vi "Sensores_LabView.vi"() -> ()   [LabVIEW 2014]
uses:
  <vilib>/LabVIEW Interface for Arduino/Type Defs/Board Type.ctl
  <vilib>/LabVIEW Interface for Arduino/Type Defs/Pin Mode.ctl
  <vilib>/LabVIEW Interface for Arduino/LabVIEW Interface for Arduino.lvlib
panel:
  out "Sensor de Movimiento":bool
  out "Sensor de temperatura":dbl(slide) scale=0.0..100.0
  out "Indicador fotoresistencia":dbl(knob) scale=0.0..100.0
  out "Sensor de Movimiento":dbl
  out "Aire acondicionado":bool
  out "Iluminacion":bool
  out "UPS":bool
  out "On / Off":bool
  in  "Iluminacion deseada":dbl
  in  "VISA resource":refnum<visa-resource-name>
  in  "stop":bool
  in  "Temperatura deseada":dbl
  # "Entradas"
  # "Salidas"
  # "Valores deseados"
  # "Información\ndel programa"
  # "Interruptores"
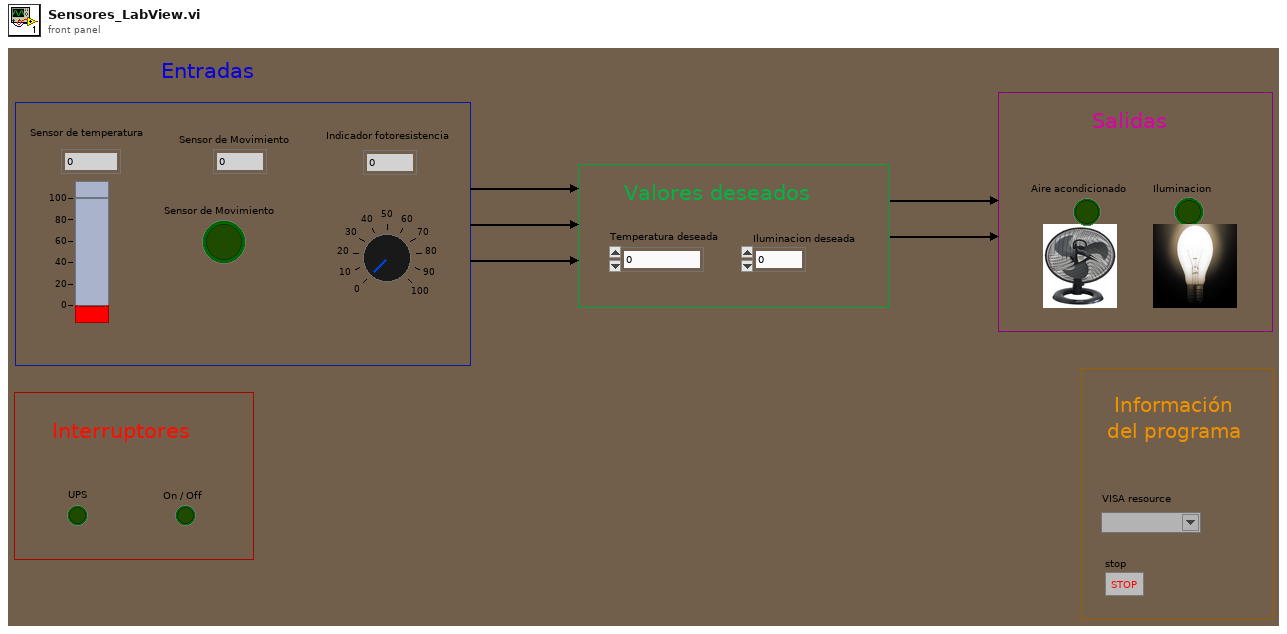
[diagram p1: front panel]
types:
  T1 = typedef "LabVIEW Interface for Arduino.lvlib/Board Type.ctl" = enum16{"Uno", "Dimuelanove w/Atmega 328", "Mega 2560"}
  T2 = typedef "LabVIEW Interface for Arduino.lvlib/Arduino Resource.ctl" = cluster{"VISA resource":refnum<visa-resource-name>, "Board Type":T1, "Connection Type":enum8{"USB / Serial"}, "Bytes Per Packet (15)":u8}
  T3 = typedef "LabVIEW Interface for Arduino.lvlib/Pin Mode.ctl" = enum8{"Input", "Output"}
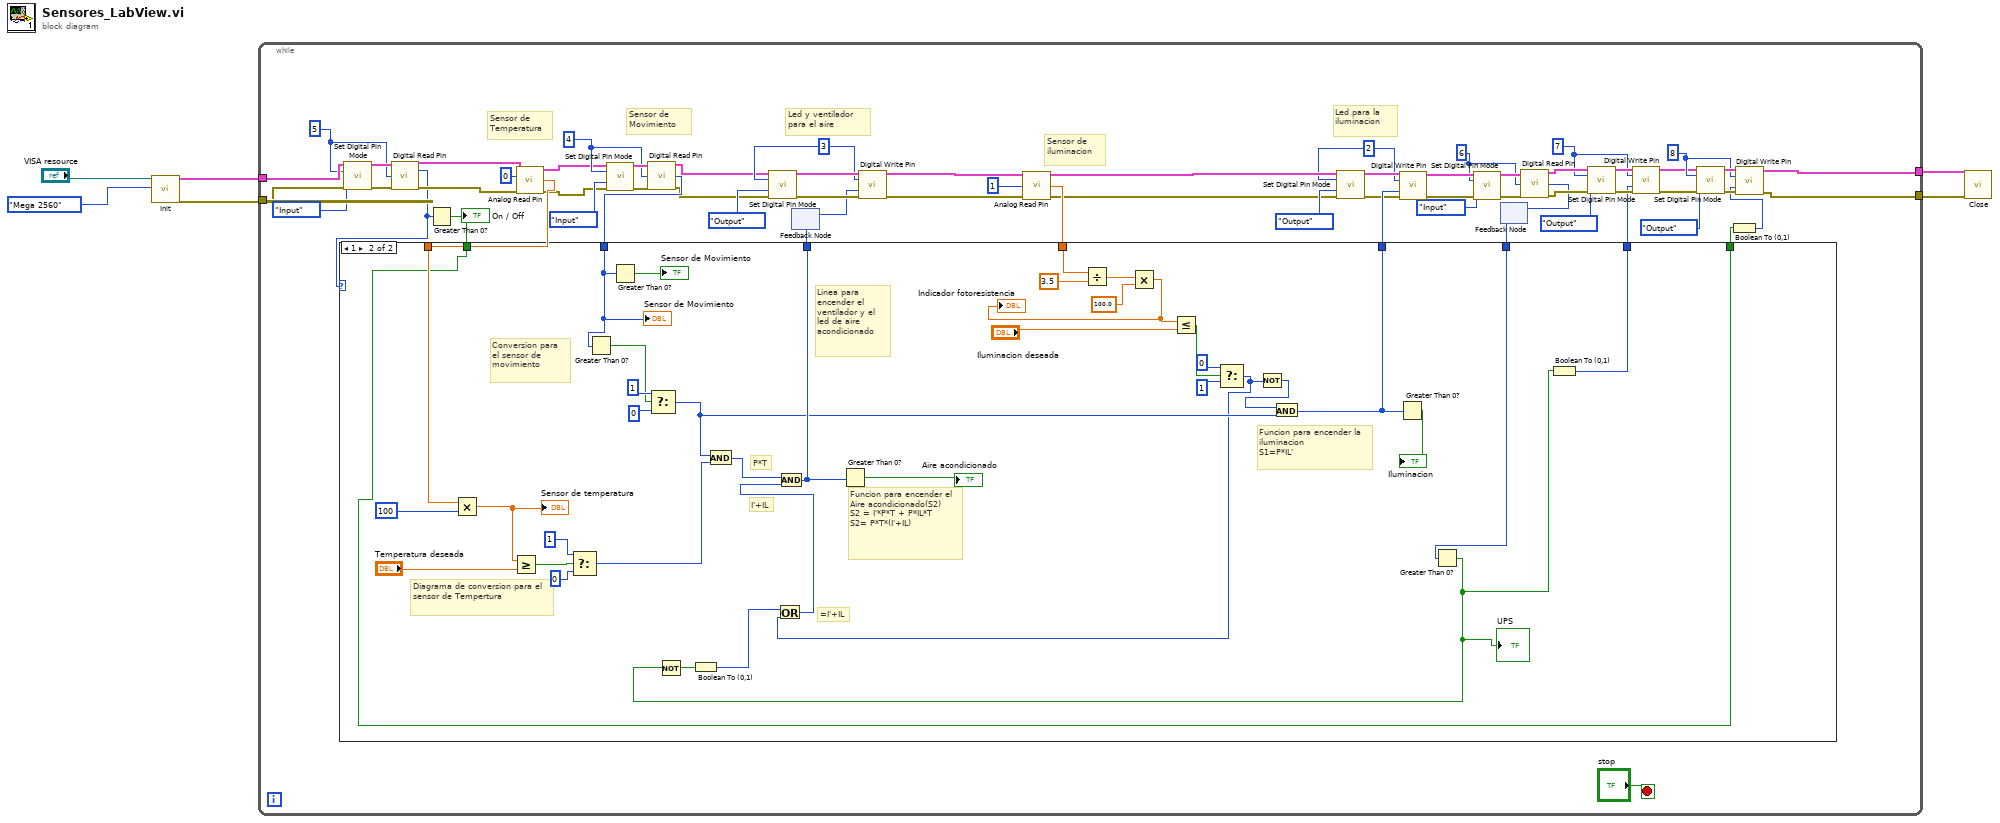
[diagram p0: block diagram]
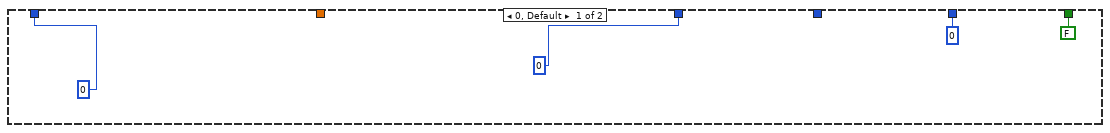
[diagram p2: hidden frame]
diagram:
  n1 = call <vilib>:"Init.vi"("VISA resource"="VISA resource", "Board Type (Uno)"=Board_Type."Mega 2560") -> ("Arduino Resource"=w6:T2, "error out"=w5:errorcluster)  [unwired: 16 in]
  n2 = while {
    tunnel: w6 -> [w37]
    tunnel: w5 -> [w36]
    tunnel: [w10] -> w3
    tunnel: [w9] -> w2
    stop <- "stop" stop-if-true
    w14 = u8 8 ("Digital I/O Pin")
    w19 = u8 7 ("Digital I/O Pin")
    w27 = u8 6 ("Digital I/O Pin")
    w35 = u8 5 ("Digital I/O Pin")
    w45 = u8 4 ("Digital I/O Pin")
    w52 = u8 2 ("Digital I/O Pin")
    w53 = u8 3 ("Digital I/O Pin")
    # "Led para la iluminacion"
    # "Led y ventilador para el aire"
    # "Sensor de Movimiento"
    # "Sensor de iluminacion"
    # "Sensor de Temperatura"
    n3 = call <vilib>:"Set Digital Pin Mode.vi"("Arduino Resource"=w37, "Digital I/O Pin"=w35, "Pin Mode (Input)"=Pin_Mode."Input", "error in"=w36) -> ("Arduino Resource"=w44:T2, "error out"=w43:errorcluster)  [unwired: 10 in]
    n4 = call <vilib>:"Digital Read Pin.vi"("Arduino Resource"=w44, "Digital I/O Pin (0)"=w35, "error in"=w43) -> ("Arduino Resource"=w41:T2, "Value"=w33:u8, "error out"=w38:errorcluster)  [unwired: 10 in]
    n5 = Greater Than 0?(x=w33) -> (x > 0?=w13:bool)
    "On / Off" <- w13
    n6 = call <vilib>:"Analog Read Pin.vi"("Arduino Resource"=w41, "Analog Input Pin (0)"=u8 0, "error in"=w38) -> ("Arduino Resource"=w39:T2, "Voltage"=w70:dbl, "error out"=w40:errorcluster)  [unwired: 10 in]
    n7 = call <vilib>:"Set Digital Pin Mode.vi"("Arduino Resource"=w39, "Digital I/O Pin"=w45, "Pin Mode (Input)"=Pin_Mode."Input", "error in"=w40) -> ("Arduino Resource"=w50:T2, "error out"=w49:errorcluster)  [unwired: 10 in]
    n8 = call <vilib>:"Digital Read Pin.vi"("Arduino Resource"=w50, "Digital I/O Pin (0)"=w45, "error in"=w49) -> ("Arduino Resource"=w47:T2, "Value"=w48:u8, "error out"=w46:errorcluster)  [unwired: 10 in]
    n9 = call <vilib>:"Set Digital Pin Mode.vi"("Arduino Resource"=w47, "Digital I/O Pin"=w53, "Pin Mode (Input)"=Pin_Mode."Output", "error in"=w46) -> ("Arduino Resource"=w65:T2, "error out"=w64:errorcluster)  [unwired: 10 in]
    n10 = feedback #1() -> (w54:i32)  [unwired: 1 in]
    n11 = call <vilib>:"Digital Write Pin.vi"("Arduino Resource"=w65, "Digital I/O Pin (0)"=w53, "Value (0)"=w54, "error in"=w64) -> ("Arduino Resource"=w61:T2, "error out"=w60:errorcluster)  [unwired: 10 in]
    n12 = call <vilib>:"Analog Read Pin.vi"("Arduino Resource"=w61, "Analog Input Pin (0)"=u8 1, "error in"=w60) -> ("Arduino Resource"=w59:T2, "Voltage"=w67:dbl, "error out"=w58:errorcluster)  [unwired: 10 in]
    n13 = call <vilib>:"Set Digital Pin Mode.vi"("Arduino Resource"=w59, "Digital I/O Pin"=w52, "Pin Mode (Input)"=Pin_Mode."Output", "error in"=w58) -> ("Arduino Resource"=w57:T2, "error out"=w56:errorcluster)  [unwired: 10 in]
    n14 = feedback #2() -> (w20:u8)  [unwired: 1 in]
    n15 = case shown="1" w33 {
      tunnel: w70 -> [_ w109]
      tunnel: w67 -> [_ w106]
      tunnel: [0 w86] -> w62
      tunnel: [0 w94] -> w55
      tunnel: w48 -> [_ w76]
      tunnel: w20 -> [_ w83]
      tunnel: [i16 0 w82] -> w18
      tunnel: w13 -> [_ w81]
      tunnel: [FALSE w81] -> w12
      frame 0, Default {
      }
      frame 1 {
        # "Funcion para encender la iluminacion\nS1=P*IL'"
        # "P*T"
        # "I'+IL"
        # "=I'+IL"
        # "Linea para encender el ventilador y el led de aire acondicionado"
        # "Funcion para encender el Aire acondicionado(S2)\nS2 = I'*P*T + P*IL*T \nS2= P*T*(I'+IL)"
        # "Conversion para el sensor de movimiento"
        # "Diagrama de conversion para el sensor de Tempertura"
        n16 = Multiply(x=w109, y=100) -> (x*y=w108:dbl)
        "Sensor de temperatura" <- w108
        n17 = Greater Or Equal?(x=w108, y="Temperatura deseada") -> (x >= y?=w104:bool)
        n18 = Select(t=1, s=w104, f=0) -> (s? t:f=w101:i32)
        n19 = Greater Than 0?(x=w76) -> (x > 0?=w84:bool)
        n20 = Greater Than 0?(x=w76) -> (x > 0?=→"Sensor de Movimiento":bool)
        n21 = Select(t=1, s=w84, f=0) -> (s? t:f=w89:i32)
        n22 = And(x=w89, y=w101) -> (x .and. y?=w96:i32)
        n23 = Divide(x=w106, y=3.5) -> (x/y=w79:dbl)
        n24 = Multiply(x=w79, y=100.0) -> (x*y=w77:dbl)
        "Indicador fotoresistencia" <- w77
        n25 = Less Or Equal?(x=w77, y="Iluminacion deseada") -> (x <= y?=w99:bool)
        n26 = Select(t=0, s=w99, f=1) -> (s? t:f=w85:i32)
        n27 = Not(x=w85) -> (.not. x?=w87:i32)
        n28 = And(x=w87, y=w89) -> (x .and. y?=w86:i32)
        n29 = Greater Than 0?(x=w86) -> (x > 0?=→"Iluminacion":bool)
        n30 = Greater Than 0?(x=w83) -> (x > 0?=w80:bool)
        "UPS" <- w80
        n31 = Not(x=w80) -> (.not. x?=w95:bool)
        n32 = Boolean To (0,1)(Boolean=w95) -> (0, 1=w88:i16)
        n33 = Or(x=w88, y=w85) -> (x .or. y?=w91:i32)
        n34 = And(x=w96, y=w91) -> (x .and. y?=w94:i32)
        n35 = Greater Than 0?(x=w94) -> (x > 0?=→"Aire acondicionado":bool)
        n36 = Boolean To (0,1)(Boolean=w80) -> (0, 1=w82:i16)
        "Sensor de Movimiento" <- w76
      }
    }
    n37 = feedback-in #1(w55) -> ()
    n38 = call <vilib>:"Digital Write Pin.vi"("Arduino Resource"=w57, "Digital I/O Pin (0)"=w52, "Value (0)"=w62, "error in"=w56) -> ("Arduino Resource"=w30:T2, "error out"=w29:errorcluster)  [unwired: 10 in]
    n39 = call <vilib>:"Set Digital Pin Mode.vi"("Arduino Resource"=w30, "Digital I/O Pin"=w27, "Pin Mode (Input)"=Pin_Mode."Input", "error in"=w29) -> ("Arduino Resource"=w32:T2, "error out"=w31:errorcluster)  [unwired: 10 in]
    n40 = call <vilib>:"Digital Read Pin.vi"("Arduino Resource"=w32, "Digital I/O Pin (0)"=w27, "error in"=w31) -> ("Arduino Resource"=w23:T2, "Value"=w21:u8, "error out"=w22:errorcluster)  [unwired: 10 in]
    n41 = feedback-in #2(w21) -> ()
    n42 = call <vilib>:"Set Digital Pin Mode.vi"("Arduino Resource"=w23, "Digital I/O Pin"=w19, "Pin Mode (Input)"=Pin_Mode."Output", "error in"=w22) -> ("Arduino Resource"=w26:T2, "error out"=w25:errorcluster)  [unwired: 10 in]
    n43 = call <vilib>:"Digital Write Pin.vi"("Arduino Resource"=w26, "Digital I/O Pin (0)"=w19, "Value (0)"=w18, "error in"=w25) -> ("Arduino Resource"=w8:T2, "error out"=w7:errorcluster)  [unwired: 10 in]
    n44 = call <vilib>:"Set Digital Pin Mode.vi"("Arduino Resource"=w8, "Digital I/O Pin"=w14, "Pin Mode (Input)"=Pin_Mode."Output", "error in"=w7) -> ("Arduino Resource"=w17:T2, "error out"=w16:errorcluster)  [unwired: 10 in]
    n45 = Boolean To (0,1)(Boolean=w12) -> (0, 1=w11:i16)
    n46 = call <vilib>:"Digital Write Pin.vi"("Arduino Resource"=w17, "Digital I/O Pin (0)"=w14, "Value (0)"=w11, "error in"=w16) -> ("Arduino Resource"=w10:T2, "error out"=w9:errorcluster)  [unwired: 10 in]
  }
  n47 = call <vilib>:"Close.vi"("Arduino Resource"=w3, "error in"=w2) -> ()  [unwired: 13 in, 1 out]
